vi "EOL Digital Input Task.vi"(8 "error in":errorcluster, 11 "path":path=path "C:/Labview Code/System/Digital Input Channel Configuration") -> (0 "error out":errorcluster, 3 "DI Task":refnum<k21>)   [LabVIEW 2018]
uses:
  <vilib>/Utility/file.llb/Read From Spreadsheet File (string).vi
  <vilib>/DAQmx/create/channels.llb/DAQmx Create Channel (DI-Digital Input).vi
panel:
  in  "子数组":string[](array[string])
  out "?":string[][](array[string])
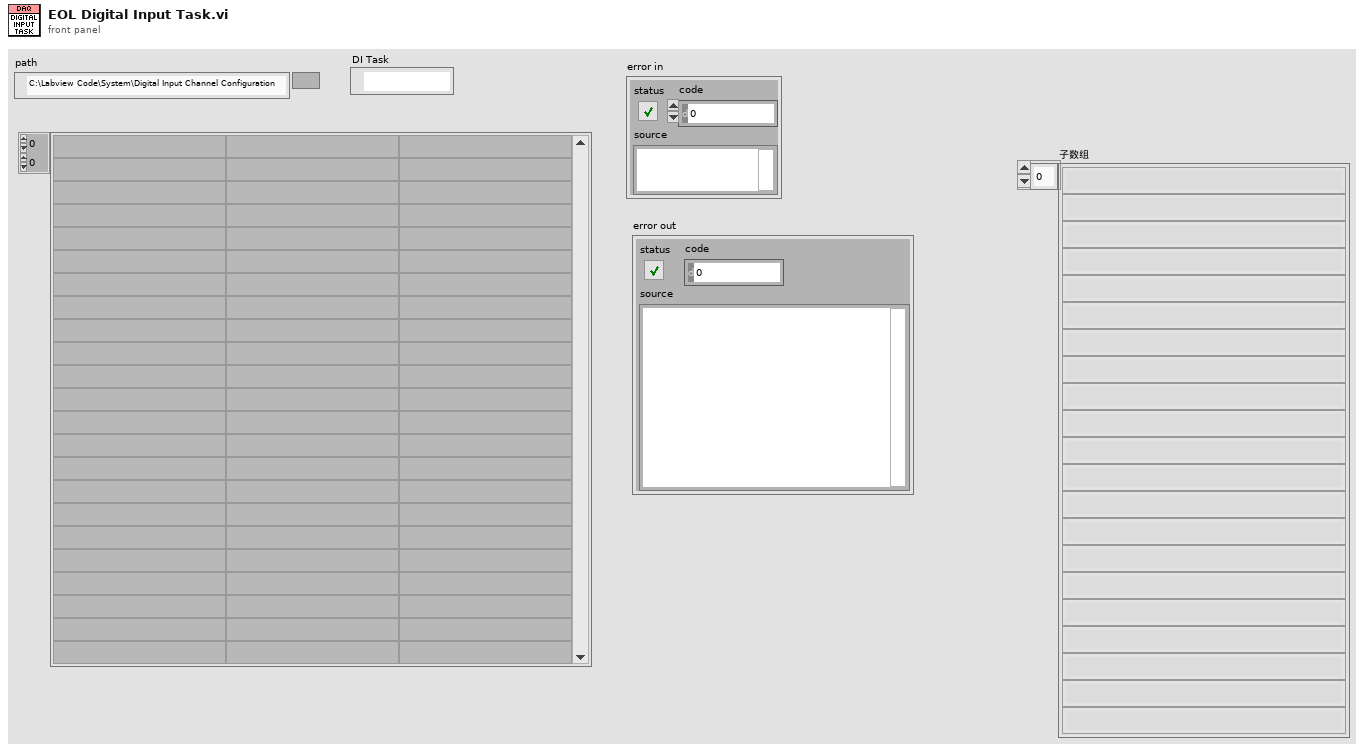
[diagram p1: front panel]
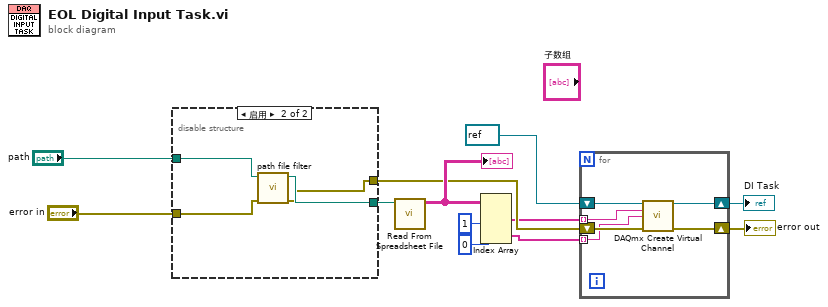
[diagram p0: block diagram]
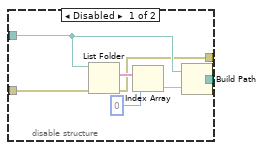
[diagram p2: hidden frame]
diagram:
  n1 = disable-structure shown="启用" {
    disable-tunnel: "path" -> [w17 w23]
    disable-tunnel: [w16 w22] -> w9
    disable-tunnel: "error in" -> [w15 w21]
    disable-tunnel: [w14 w20] -> w7
    frame Disabled {
      n2 = List Folder(path=w17, error in=w15) -> (filenames=w19:string[], error out=w14:errorcluster)  [unwired: 2 in, 2 out]
      n3 = Index Array(array=w19, index=0 ("索引")) -> (element=w18:string)
      n4 = Build Path(base path=w17, name or relative path=w18) -> (appended path=w16:path)
    }
    frame Enabled {
      n5 = call "path file filter.vi"("Sys Error In"=w21, "path"=w23) -> ("错误输出"=w20:errorcluster, "File path"=w22:path)  [unwired: 8 in]
    }
  }
  n6 = call-poly <vilib>:"Read From Spreadsheet File.vi"("file path (dialog if empty)"=w9) -> ("all rows"=w12:string[][])  [unwired: 6 in, 4 out]
  "?" <- w12
  n7 = Index Array(array=w12, index (col) #1=1 ("disabled index (col)"), index (col) #2=0 ("索引 (列)")) -> (element #1=w2:string[], element #2=w1:string[])  [unwired: 2 in]
  n8 = for {
    tunnel: w2 -> [w27] mode=indexing
    shift-right: [w29] -> w5
    shift-left: refnum<k21> refnum ("task out") -> [w28]
    shift-right: [w26] -> w6
    shift-left: w7 -> [w25]
    tunnel: w1 -> [w24] mode=indexing
    n9 = call-poly <vilib>:"DAQmx Create Virtual Channel.vi"("task in"=w28, "lines"=w27, "name to assign"=w24, "error in"=w25) -> ("task out"=w29:refnum<k21>, "error out"=w26:errorcluster)  [unwired: 10 in]
  }
  "DI Task" <- w5
  "error out" <- w6
